vi "方向机测试台.vi"() -> ()   [LabVIEW 2015]
doc: "该连续测量范例项目在队列消息处理器模板的基础上实现。\n\n事件处理循环负责按用户界面操作生成对应的消息。\n\n消息处理循环负责对事件处理循环或其他消息生成的消息进行处理。其中还包括用于采集和记录消息处理循环的子VI，以及用于更新图表的循环。"
uses:
  support/Message Queue/Enqueue Message (Single).vi
  <vilib>/Utility/error.llb/Error Cluster From Error Code.vi
  <vilib>/ErrorRing/Error Ring.xnode
  support/User Event - Stop/User Event - Stop.lvlib
  support/Message Queue/Message Queue.lvlib
  Settings/Settings.lvlib
panel:
  in  "内泄漏":bool
  in  "设置":bool
  in  "力特性":bool
  in  "功能":bool
  in  "湿退回":bool
  in  "干退回":bool
  in  "湿啮合":bool
  in  "干啮合":bool
  # "方向机测试台"
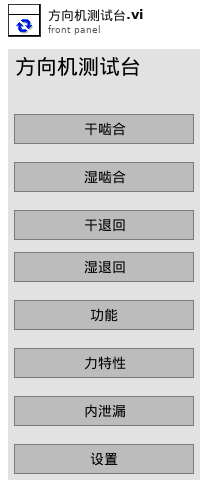
[diagram p1: front panel]
types:
  T1 = typedef "Settings.lvlib/Settings.ctl" = cluster{"Hardware Configuration":T2, "Logging Configuration":T3, "Action Configuration":T4}
  T2 = typedef "Acquisition.lvlib/Hardware Configuration.ctl" = cluster{"电压读取设置":cluster{"DAQmx Channel":tag, "Max Input":dbl, "Min Input":dbl, "Sample Rate":dbl, "Sample Number":i32, "DAQmx Task":refnum<k21>, "device in":tag}, "角度传感器设置":cluster{"counter":tag, "units":i32, "分辨率":i32, "初始角度":dbl, "DecodingType":i32, "A相端口":tag, "B相端口":tag, "task in":refnum<k21>}}
  T3 = typedef "Logging.lvlib/Logging Configuration.ctl" = cluster{"Log File Base Path":path, "电压传感器转换率":dbl[], "电压传感器本底":dbl[], "测试模式是否需要保存数据？":bool}
  T4 = typedef "Action.lvlib/Hardware Configuration.ctl" = cluster{"PLC设置":T5, "动作设置":T6, "电机设置":T10, "所有测试电机转动逻辑":T11}
  T5 = typedef "Action.lvlib/PLC设置.ctl" = cluster{"ActLogicalStationNumber":i32, "ActUtlType":refnum<k7>}
  T6 = typedef "Action.lvlib/动作设置.ctl" = cluster{"自动跳法测试动作":T7, "其他动作":T9}
  T7 = typedef "Action.lvlib/自动调阀测试动作设置.ctl" = cluster{"夹紧阀总":T8, "夹紧/松阀芯":T8, "方向机供油":T8, "扭杆紧/松":T8, "电机使能":T8, "内泄漏开":T8, "内泄漏停":T8, "数控钻孔启动":T8, "托起缸上":T8, "托起缸下":T8, "内泄漏放油":T8, "读取开始按钮":T8, "读取压销启动":T8, "读取压销完成":T8, "放松阀总":T8, "卡盘松紧":T8}
  T8 = typedef "Action.lvlib/PLC控制指令.ctl" = cluster{"变量类型":u32, "PLC地址":i32, "size":i32, "写入数据(写入时有效)":i16}
  T9 = typedef "Action.lvlib/其他动作设置 .ctl" = cluster{"其他指令1":T8, "其他指令2":T8, "其他指令3":T8, "其他指令4":T8, "其他指令5":T8}
  T10 = typedef "Action.lvlib/电机控制设置.ctl" = cluster{"counter":tag, "方向端口":tag, "当前方向":bool, "频率":dbl, "DAQmx Task":refnum<k21>}
  T11 = typedef "Action.lvlib/所有测试电机转动逻辑.ctl" = cluster{"啮合测试电机转动逻辑":T12, "退回测试电机转动逻辑":T12, "功能测试电机转动逻辑":T12, "力特性测试电机转动逻辑":T12, "自动调阀测试分中电机转动逻辑":T12, "自动调阀测试对中电机转动逻辑":T12, "内泄漏电机转动逻辑":T12}
  T12 = typedef "Action.lvlib/电机转动逻辑1.ctl" = cluster{"反转判断条件1":T13, "停止判断条件1":T14}
  T13 = typedef "Action.lvlib/反转判断条件1.ctl" = cluster{"传感器序号":i32, "条件":enum16{"小于", "大于", "等于"}, "值":dbl, "条件判断时间间隔":i32}
  T14 = typedef "Action.lvlib/停止判断条件1.ctl" = cluster{"传感器序号":i32, "正转/反转":enum16{"正转", "反转"}, "反转次数":i32, "停止角度":dbl, "停止误差范围":dbl}
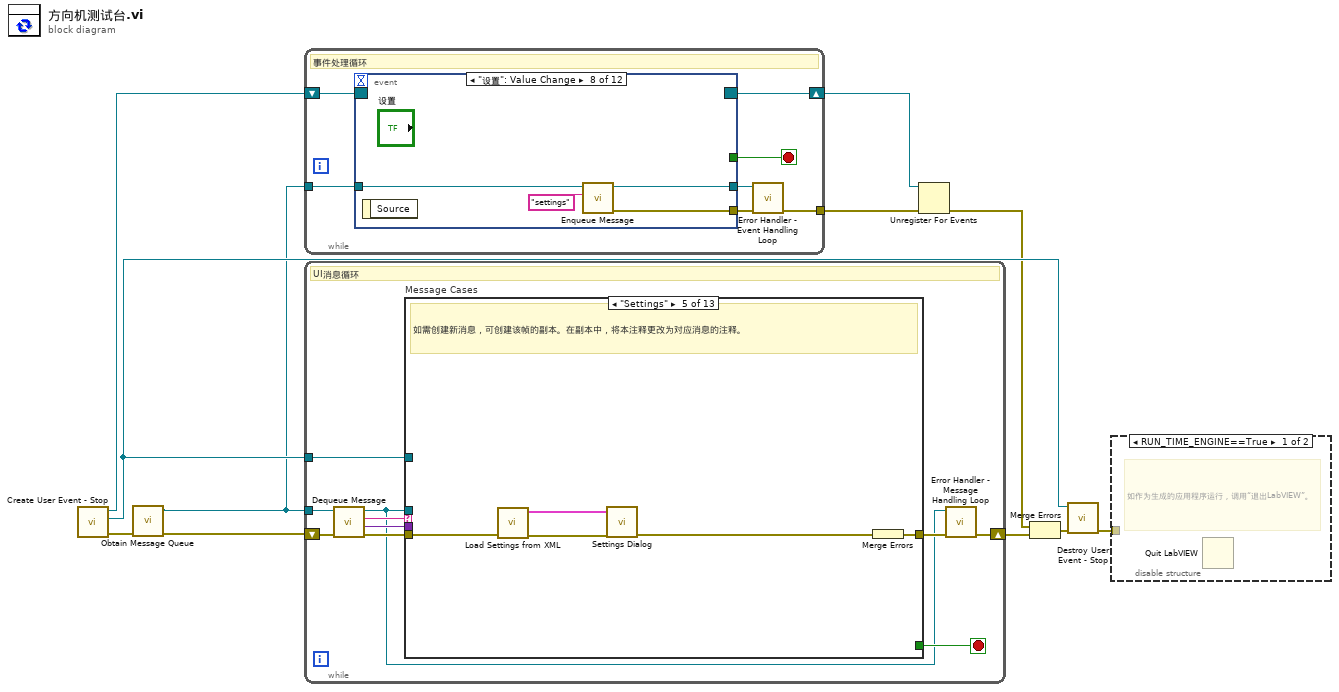
[diagram p0: block diagram]
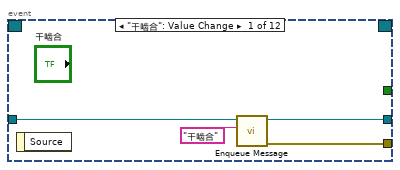
[diagram p3: hidden frame]
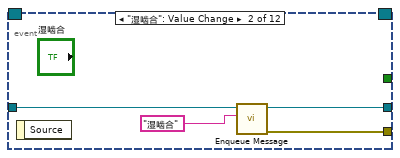
[diagram p4: hidden frame]
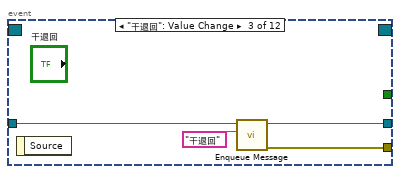
[diagram p5: hidden frame]
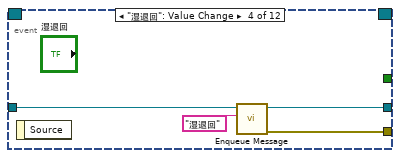
[diagram p6: hidden frame]
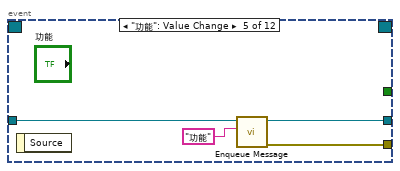
[diagram p7: hidden frame]
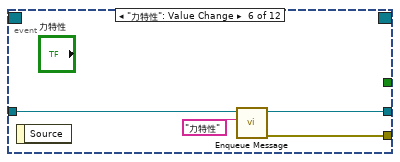
[diagram p8: hidden frame]
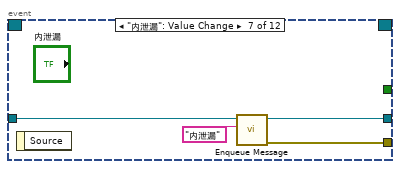
[diagram p9: hidden frame]
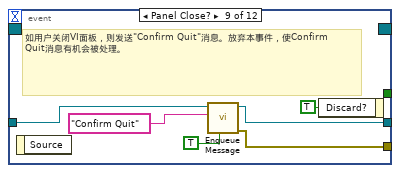
[diagram p10: hidden frame]
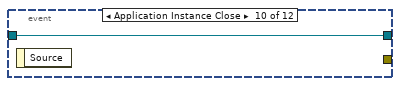
[diagram p11: hidden frame]
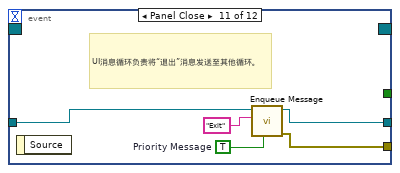
[diagram p12: hidden frame]
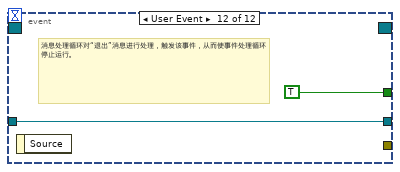
[diagram p13: hidden frame]
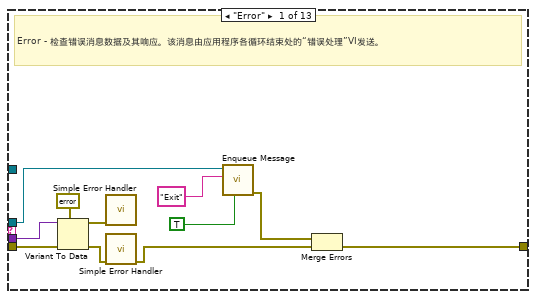
[diagram p14: hidden frame]
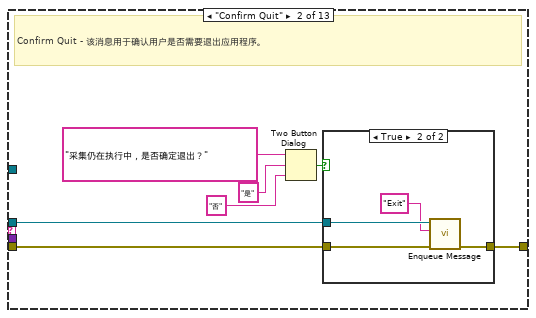
[diagram p15: hidden frame]
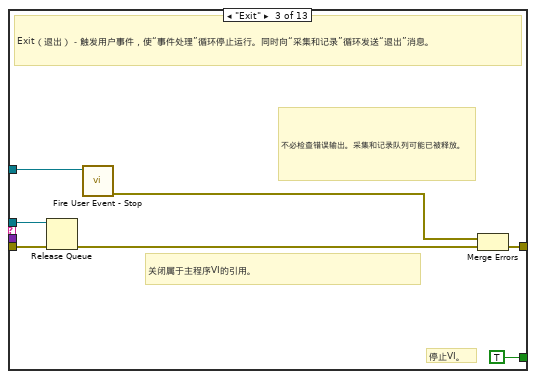
[diagram p17: hidden frame]
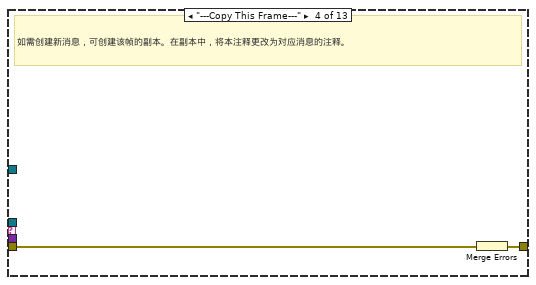
[diagram p18: hidden frame]
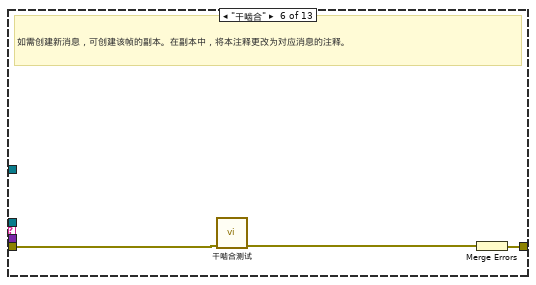
[diagram p19: hidden frame]
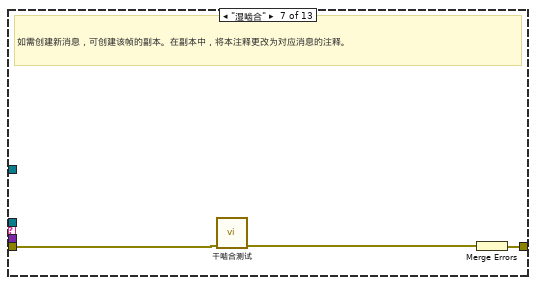
[diagram p20: hidden frame]
diagram:
  n1 = call "Create User Event - Stop.vi"() -> ("error out"=w3:errorcluster, "User Event - Stop"=w7:refnum<user-event>, "Stop Event Registration Refnum"=w8:refnum<event-registration>)  [unwired: 9 in]
  n2 = call "Obtain Message Queue.vi"("error in (no error)"=w3) -> ("error out"=w1:errorcluster, "Message Queue"=w2:refnum<queue>)  [unwired: 9 in]
  n3 = while {
    tunnel: w2 -> [w17]
    tunnel: [w12] -> w10
    shift-right: [w16] -> w5
    shift-left: w8 -> [w18]
    stop <- w15 stop-if-true
    # "事件处理循环"
    n4 = event shown="[7] \"设置\": Value Change" {
      selector: w18 -> [_ _ _ _ _ _ _ _ _ _ _ _]
      dyn-events: [_ _ _ _ _ _ _ _ _ _ _ _] -> w16
      timeout: _ -> [_ _ _ _ _ _ _ _ _ _ _ _]
      tunnel: [_ _ _ _ _ _ _ _ _ _ _ TRUE ("Discard?")] -> w15
      tunnel: w17 -> [w20 w25 w29 w33 w37 w41 w45 w49 w56 w57 w59 w63]
      tunnel: [w22 w24 w28 w32 w36 w40 w44 w48 w51 _ w62 _] -> w13
      tunnel: [w19 w23 w27 w31 w35 w39 w43 w47 w52 w57 w58 w63] -> w14
      event "干啮合": Value Change {
        n5 = event-data() -> ()  [unwired: 1 in, 1 out]
        n6 = call-poly "Enqueue Message.vi"("Message"="干啮合", "Message Queue"=w20) -> ("error out"=w22:errorcluster, "dup Message Queue"=w19:refnum<queue>)  [unwired: 8 in]
      }
      event "湿啮合": Value Change {
        n7 = event-data() -> ()  [unwired: 1 in, 1 out]
        n8 = call-poly "Enqueue Message.vi"("Message"="湿啮合", "Message Queue"=w25) -> ("error out"=w24:errorcluster, "dup Message Queue"=w23:refnum<queue>)  [unwired: 8 in]
      }
      event "干退回": Value Change {
        n9 = event-data() -> ()  [unwired: 1 in, 1 out]
        n10 = call-poly "Enqueue Message.vi"("Message"="干退回", "Message Queue"=w29) -> ("error out"=w28:errorcluster, "dup Message Queue"=w27:refnum<queue>)  [unwired: 8 in]
      }
      event "湿退回": Value Change {
        n11 = event-data() -> ()  [unwired: 1 in, 1 out]
        n12 = call-poly "Enqueue Message.vi"("Message"="湿退回", "Message Queue"=w33) -> ("error out"=w32:errorcluster, "dup Message Queue"=w31:refnum<queue>)  [unwired: 8 in]
      }
      event "功能": Value Change {
        n13 = event-data() -> ()  [unwired: 1 in, 1 out]
        n14 = call-poly "Enqueue Message.vi"("Message"="功能", "Message Queue"=w37) -> ("error out"=w36:errorcluster, "dup Message Queue"=w35:refnum<queue>)  [unwired: 8 in]
      }
      event "力特性": Value Change {
        n15 = event-data() -> ()  [unwired: 1 in, 1 out]
        n16 = call-poly "Enqueue Message.vi"("Message"="力特性", "Message Queue"=w41) -> ("error out"=w40:errorcluster, "dup Message Queue"=w39:refnum<queue>)  [unwired: 8 in]
      }
      event "内泄漏": Value Change {
        n17 = event-data() -> ()  [unwired: 1 in, 1 out]
        n18 = call-poly "Enqueue Message.vi"("Message"="内泄漏", "Message Queue"=w45) -> ("error out"=w44:errorcluster, "dup Message Queue"=w43:refnum<queue>)  [unwired: 8 in]
      }
      event "设置": Value Change {
        n19 = event-data() -> ()  [unwired: 1 in, 1 out]
        n20 = call-poly "Enqueue Message.vi"("Message"="settings", "Message Queue"=w49) -> ("error out"=w48:errorcluster, "dup Message Queue"=w47:refnum<queue>)  [unwired: 8 in]
      }
      event Panel Close? {
        # "如用户关闭VI面板，则发送\"Confirm Quit\"消息。放弃本事件，使Confirm Quit消息有机会被处理。"
        n21 = event-data() -> ()  [unwired: 1 in, 1 out]
        n22 = call-poly "Enqueue Message.vi"("Priority Message? (F)"=TRUE, "Message"="Confirm Quit", "Message Queue"=w56) -> ("error out"=w51:errorcluster, "dup Message Queue"=w52:refnum<queue>)  [unwired: 7 in]
        n23 = event-data("Discard?"=TRUE) -> ()  [unwired: 1 in, 1 out]
      }
      event Application Instance Close {
        n24 = event-data() -> ()  [unwired: 1 in, 1 out]
      }
      event Panel Close {
        w60 = TRUE  # Priority Message
        # "UI消息循环负责将“退出”消息发送至其他循环。"
        n25 = event-data() -> ()  [unwired: 1 in, 1 out]
        n26 = call-poly "Enqueue Message.vi"("Priority Message? (F)"=w60, "Message"="Exit", "Message Queue"=w59) -> ("error out"=w62:errorcluster, "dup Message Queue"=w58:refnum<queue>)  [unwired: 7 in]
      }
      event User Event {
        # "消息处理循环对“退出”消息进行处理，触发该事件，从而使事件处理循环停止运行。"
        n27 = event-data() -> ()  [unwired: 1 in, 1 out]
      }
    }
    n28 = call "Error Handler - Event Handling Loop.vi"("error in (no error)"=w13, "Message Queue"=w14) -> ("dup error in"=w12:errorcluster)  [unwired: 8 in, 1 out]
  }
  n29 = while {
    tunnel: w2 -> [w68]
    tunnel: w7 -> [w73]
    shift-right: [w66] -> w11
    shift-left: w1 -> [w72]
    stop <- w74 stop-if-true
    # "UI消息循环"
    n30 = call "Dequeue Message.vi"("error in (no error)"=w72, "Message Queue"=w68) -> ("error out"=w71:errorcluster, "Message Data"=w69:variant, "Message"=w70:string, "dup Message Queue"=w65:refnum<queue>)  [unwired: 6 in]
    n31 = case "Message Cases" shown="\"Settings\"" w70 {
      selector: w70 -> [_ _ _ _ _ _ _ _ _ _ _ _ w133]
      tunnel: w65 -> [w81 w92 w99 _ _ _ _ _ _ _ _ _ _]
      tunnel: w71 -> [w85 w91 w102 w106 w109 w113 w116 w119 w122 w125 w128 w131 _]
      tunnel: [w77 w90 w103 w105 w111 w114 w117 w120 w123 w126 w129 w132 w134] -> w67
      tunnel: [_ _ TRUE _ _ _ _ _ _ _ _ _ _] -> w74
      tunnel: w69 -> [w84 _ _ _ _ _ _ _ _ _ _ _ _]
      tunnel: w73 -> [_ _ w101 _ _ _ _ _ _ _ _ _ _]
      frame "Error" {
        # "Error - 检查错误消息数据及其响应。该消息由应用程序各循环结束处的“错误处理”VI发送。"
        n32 = Variant To Data(error in=w85, type=errorcluster {"status"=FALSE, "code"=0, "source"=""} ("error out"), Variant=w84) -> (data=w82:errorcluster, error out=w76:errorcluster)
        n33 = call <vilib>:"Simple Error Handler.vi"("error in (no error)"=w82) -> ()  [unwired: 4 in, 5 out]
        n34 = call <vilib>:"Simple Error Handler.vi"("error in (no error)"=w76) -> ("error out"=w75:errorcluster)  [unwired: 4 in, 4 out]
        n35 = call-poly "Enqueue Message.vi"("Priority Message? (F)"=TRUE, "Message"="Exit", "Message Queue"=w81) -> ("error out"=w78:errorcluster)  [unwired: 7 in, 1 out]
        n36 = Merge Errors(w78, w75) -> (w77:errorcluster)
      }
      frame "Confirm Quit" {
        # "Confirm Quit - 该消息用于确认用户是否需要退出应用程序。"
        n37 = Two Button Dialog(message="采集仍在执行中，是否确定退出？" ("Confirm Quit Message"), 1:"否" ("No"), 2:"是" ("Yes")) -> (T button?=w86:bool)
        n38 = case shown="True" w86 {
          tunnel: w92 -> [_ w97]
          tunnel: w91 -> [w93 w96]
          tunnel: [w93 w95] -> w90
          frame False {
          }
          frame True {
            n39 = call-poly "Enqueue Message.vi"("error in (no error)"=w96, "Message"="Exit", "Message Queue"=w97) -> ("error out"=w95:errorcluster)  [unwired: 7 in, 1 out]
          }
        }
      }
      frame "Exit" {
        # "不必检查错误输出。采集和记录队列可能已被释放。"
        # "关闭属于主程序VI的引用。"
        # "停止VI。"
        # "Exit（退出）－触发用户事件，使“事件处理”循环停止运行。同时向“采集和记录”循环发送“退出”消息。"
        n40 = Release Queue(queue=w99, error in (no error)=w102) -> (error out=w98:errorcluster)  [unwired: 1 in, 2 out]
        n41 = call "Fire User Event - Stop.vi"("User Event - Stop"=w101) -> ("error out"=w100:errorcluster)  [unwired: 10 in]
        n42 = Merge Errors(w100, w98) -> (w103:errorcluster)
      }
      frame "---Copy This Frame---" {
        # "如需创建新消息，可创建该帧的副本。在副本中，将本注释更改为对应消息的注释。"
        n43 = Merge Errors(w106) -> (w105:errorcluster)
      }
      frame "Settings" {
        # "如需创建新消息，可创建该帧的副本。在副本中，将本注释更改为对应消息的注释。"
        n44 = call "Load Settings from XML.vi"("error in (no error)"=w109) -> ("error out"=w108:errorcluster, "Settings out"=w107:T1)  [unwired: 9 in]
        n45 = call "Settings Dialog.vi"("error in (no error)"=w108, "Settings in"=w107) -> ("error out"=w110:errorcluster)  [unwired: 6 in, 3 out]
        n46 = Merge Errors(w110) -> (w111:errorcluster)
      }
      frame "干啮合" {
        # "如需创建新消息，可创建该帧的副本。在副本中，将本注释更改为对应消息的注释。"
        n47 = call "干啮合测试.vi"("error in (no error)"=w113) -> ("error out"=w112:errorcluster)  [unwired: 10 in]
        n48 = Merge Errors(w112) -> (w114:errorcluster)
      }
      frame "湿啮合" {
        # "如需创建新消息，可创建该帧的副本。在副本中，将本注释更改为对应消息的注释。"
        n49 = call "干啮合测试.vi"("error in (no error)"=w116) -> ("error out"=w115:errorcluster)  [unwired: 10 in]
        n50 = Merge Errors(w115) -> (w117:errorcluster)
      }
      frame "干退回" {
        # "如需创建新消息，可创建该帧的副本。在副本中，将本注释更改为对应消息的注释。"
        n51 = call "干退回测试.vi"("error in (no error)"=w119) -> ("error out"=w118:errorcluster)  [unwired: 10 in]
        n52 = Merge Errors(w118) -> (w120:errorcluster)
      }
      frame "湿退回" {
        # "如需创建新消息，可创建该帧的副本。在副本中，将本注释更改为对应消息的注释。"
        n53 = call "干退回测试.vi"("error in (no error)"=w122) -> ("error out"=w121:errorcluster)  [unwired: 10 in]
        n54 = Merge Errors(w121) -> (w123:errorcluster)
      }
      frame "功能" {
        # "如需创建新消息，可创建该帧的副本。在副本中，将本注释更改为对应消息的注释。"
        n55 = call "功能测试.vi"("error in (no error)"=w125) -> ("error out"=w124:errorcluster)  [unwired: 10 in]
        n56 = Merge Errors(w124) -> (w126:errorcluster)
      }
      frame "力特性" {
        # "如需创建新消息，可创建该帧的副本。在副本中，将本注释更改为对应消息的注释。"
        n57 = call "力特性测试.vi"("error in (no error)"=w128) -> ("error out"=w127:errorcluster)  [unwired: 10 in]
        n58 = Merge Errors(w127) -> (w129:errorcluster)
      }
      frame "内泄漏" {
        # "如需创建新消息，可创建该帧的副本。在副本中，将本注释更改为对应消息的注释。"
        n59 = call "内泄漏.vi"("error in (no error)"=w131) -> ("error out"=w130:errorcluster)  [unwired: 10 in]
        n60 = Merge Errors(w130) -> (w132:errorcluster)
      }
      frame Default {
        # "如得到的消息未经任何分支定义，则运行“默认”分支。输出程序错误。"
        n61 = xnode "Error Ring"("parameter 0"=w133) -> ("error out"=w134:errorcluster)
      }
    }
    n62 = call "Error Handler - Message Handling Loop.vi"("error in (no error)"=w67, "Message Queue"=w65) -> ("dup error in"=w66:errorcluster)  [unwired: 8 in, 1 out]
  }
  n63 = Unregister For Events(event registration refnum=w5, error in=w10) -> (error out=w6:errorcluster)
  n64 = Merge Errors(w6, w11) -> (w9:errorcluster)
  n65 = call "Destroy User Event - Stop.vi"("error in (no error)"=w9, "User Event - Stop"=w7) -> ("error out"=w4:errorcluster)  [unwired: 9 in]
  n66 = disable-structure shown="RUN_TIME_ENGINE==True" {
    disable-tunnel: w4 -> [_ _]
    frame condition #0 {
      # "如作为生成的应用程序运行，调用“退出LabVIEW”。"
      n67 = Quit LabVIEW() -> ()  [unwired: 1 in]
    }
    frame condition #1 (active) {
    }
  }
